vi "Module Timeout--constant.vi"(6 "Module ID":i32=-1) -> (3 "Module Timeout":i32)   [LabVIEW 2020, in "hse-db.lvlib" / "DB_CONNECTOR.lvlib"]
doc: "A module-wide common value to use as the timeout for various synchronization actions.\n____\nHAMPEL SOFTWARE ENGINEERING v1.4.0 (2023-12-19 09:52)"
uses:
  DB_CONNECTOR.lvlib
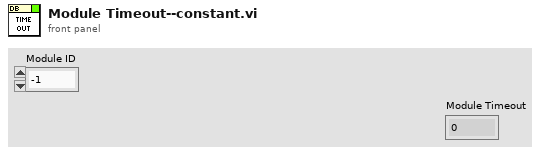
[diagram p1: front panel]
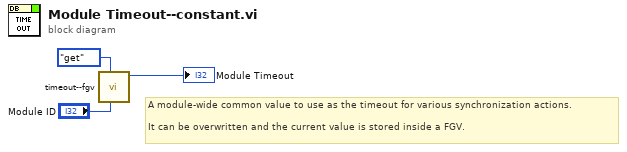
[diagram p0: block diagram]
diagram:
  # "A module-wide common value to use as the timeout for various synchronization actions.\n\nIt can be overwritten and the current value is stored inside a FGV."
  n1 = call "timeout--fgv.vi"("Module ID"="Module ID", "Action"=enum16{"set", "get"}."get") -> ("Module Timeout out"=→"Module Timeout":i32)  [unwired: 9 in]
